vi "people_count.vi"() -> (0 "data out":string)   [LabVIEW 2024]
uses:
  94cd4111-eafa-445e-ad6f-57004a1cda30.vi
panel:
  out "name":string
  out "address":u32
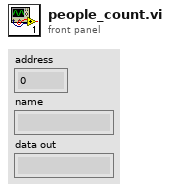
[diagram p1: front panel]
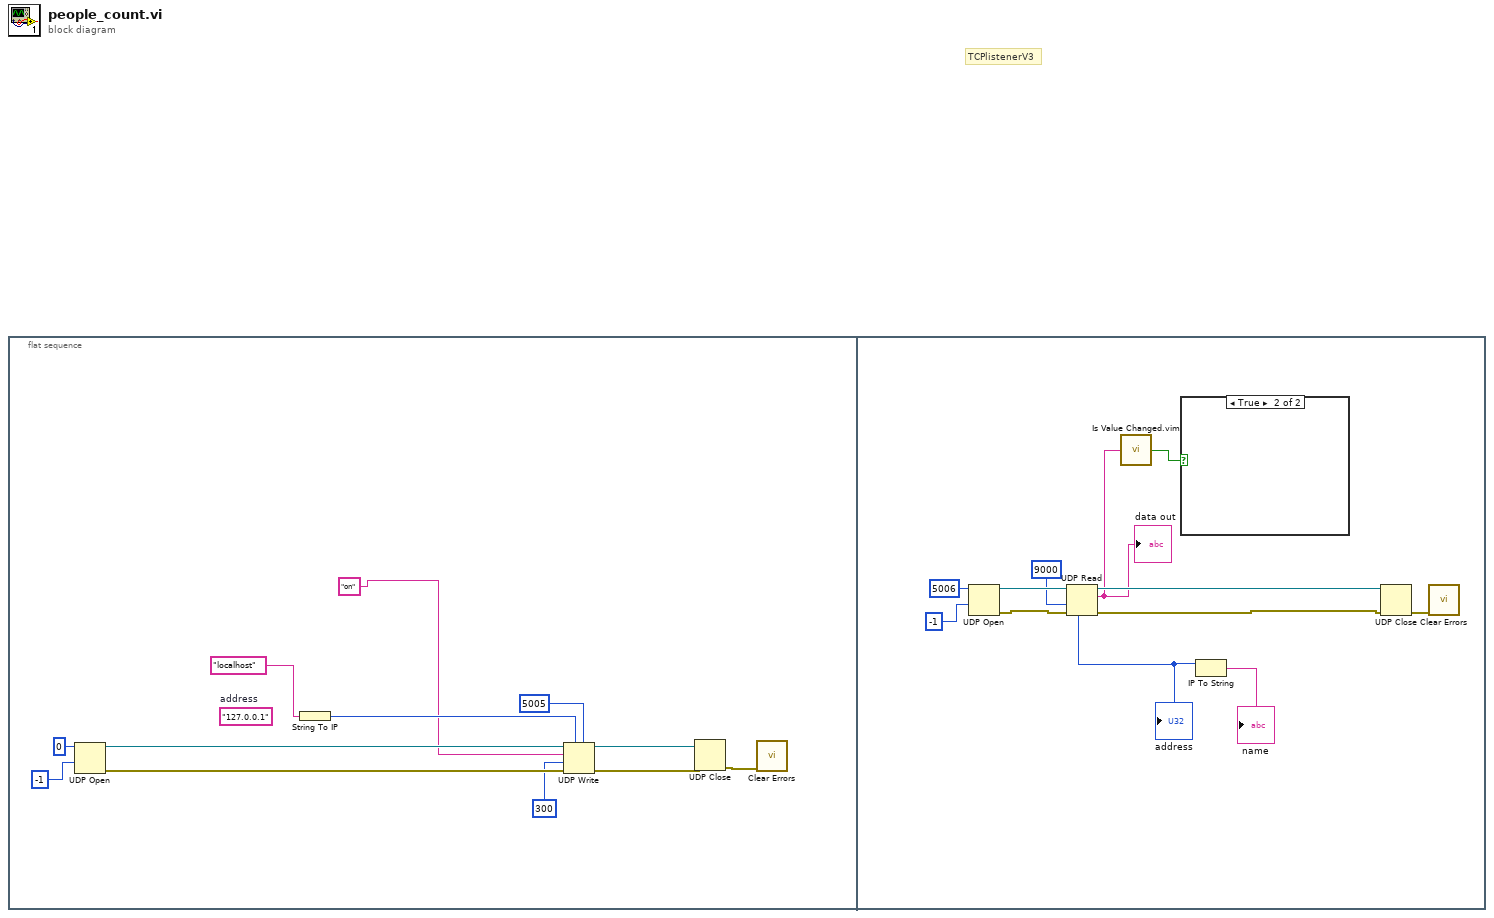
[diagram p0: block diagram]
diagram:
  # "TCPlistenerV3"
  n1 = flat-sequence {
    frame #0 {
      (unwired) "127.0.0.1"  # address
      n2 = UDP Open(9:-1 ("timeout ms (60000)"), 11:u16 0 ("port")) -> (port=w9:refnum<k16>, 0:w10:errorcluster)  [unwired: 3 in, 1 out]
      n3 = String To IP(1:"localhost" ("address")) -> (0:w4:u32)
      n4 = UDP Write(address=w4, port or service name=u16 5005, connection ID=w9, data in="on", 8:w10, 9:300 ("timeout ms (25000)")) -> (error out=w7:errorcluster, 3:w6:refnum<k16>)
      n5 = UDP Close(connection ID=w6, 8:w7) -> (error out=w8:errorcluster)  [unwired: 1 out]
      n6 = call <vilib>:"Clear Errors.vi"("error in (no error)"=w8) -> ()  [unwired: 5 in, 2 out]
    }
    frame #1 {
      n7 = UDP Open(9:-1 ("timeout ms (60000)"), 11:u16 5006 ("port")) -> (port=w20:refnum<k16>, 0:w21:errorcluster)  [unwired: 3 in, 1 out]
      n8 = UDP Read(connection ID=w20, timeout ms (25000)=9000, 8:w21) -> (data out=w13:string, error out=w24:errorcluster, 3:w23:refnum<k16>, 6:w17:u32)  [unwired: 1 in, 1 out]
      "address" <- w17
      "data out" <- w13
      n9 = call "Is Value Changed.vim"("value"=w13) -> ("changed or first call?"=w14:bool)
      n10 = case shown="True" w14 {
        frame False {
        }
        frame True {
        }
      }
      n11 = IP To String(2:w17) -> (0:→"name":string)  [unwired: 1 in]
      n12 = UDP Close(connection ID=w23, 8:w24) -> (error out=w22:errorcluster)  [unwired: 1 out]
      n13 = call <vilib>:"Clear Errors.vi"("error in (no error)"=w22) -> ()  [unwired: 5 in, 2 out]
    }
  }
